vi "subsciber 1.vi"() -> ()   [LabVIEW 2022 SP3]
uses:
  Global 1.vi
panel:
  out "String":string
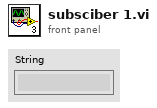
[diagram p1: front panel]
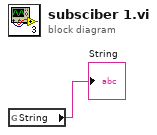
[diagram p0: block diagram]
diagram:
  n1 = global read "Global 1.vi" "String"() -> (→"String":string)
